vi "Fetch Multiple Record Multiple Channel (I16).vi"(5 "FIFO Type":enum16{"FPGA to Host FIFO (U64)", "Generic"}(ring), 7 "Timeout (s)":i32=5, 8 "error in":errorcluster, 10 "Records to Fetch":i32, 11 "FPGA VI Reference In":refnum<k20>) -> (0 "error out":errorcluster, 2 "Acquired Data":i16[][](array[numeric]), 3 "FPGA VI Reference Out":refnum<k20>, 4 "Elements Remaining":u32)   [LabVIEW 2011]
uses:
  <userlib>/FlexRIO Host Library/FlexRIO Host API/Acquire/Fetch/Fetch Acquired Data (U64).vi
  <vilib>/Utility/error.llb/Error Cluster From Error Code.vi
  <vilib>/rvi/errors/niLvFpgaAdjustHostInterfaceError.vi
  <vilib>/rvi/interface/nirviReadWriteControl/nirviReadWriteControl.xnode
  NiFpgaLv.dll
  <vilib>/rvi/interface/Simulation/niFpgaSimulationCallBeginRW.vi
  <userlib>/FlexRIO Host Library/FlexRIO Host Library (User).lvlib
  <userlib>/FlexRIO Host Library/FlexRIO Host API/Utility/memnoncopy.dll
panel:
  out "Data Acquired":i16[](array[numeric])
  out "Dummy Data":i16[](array[numeric])
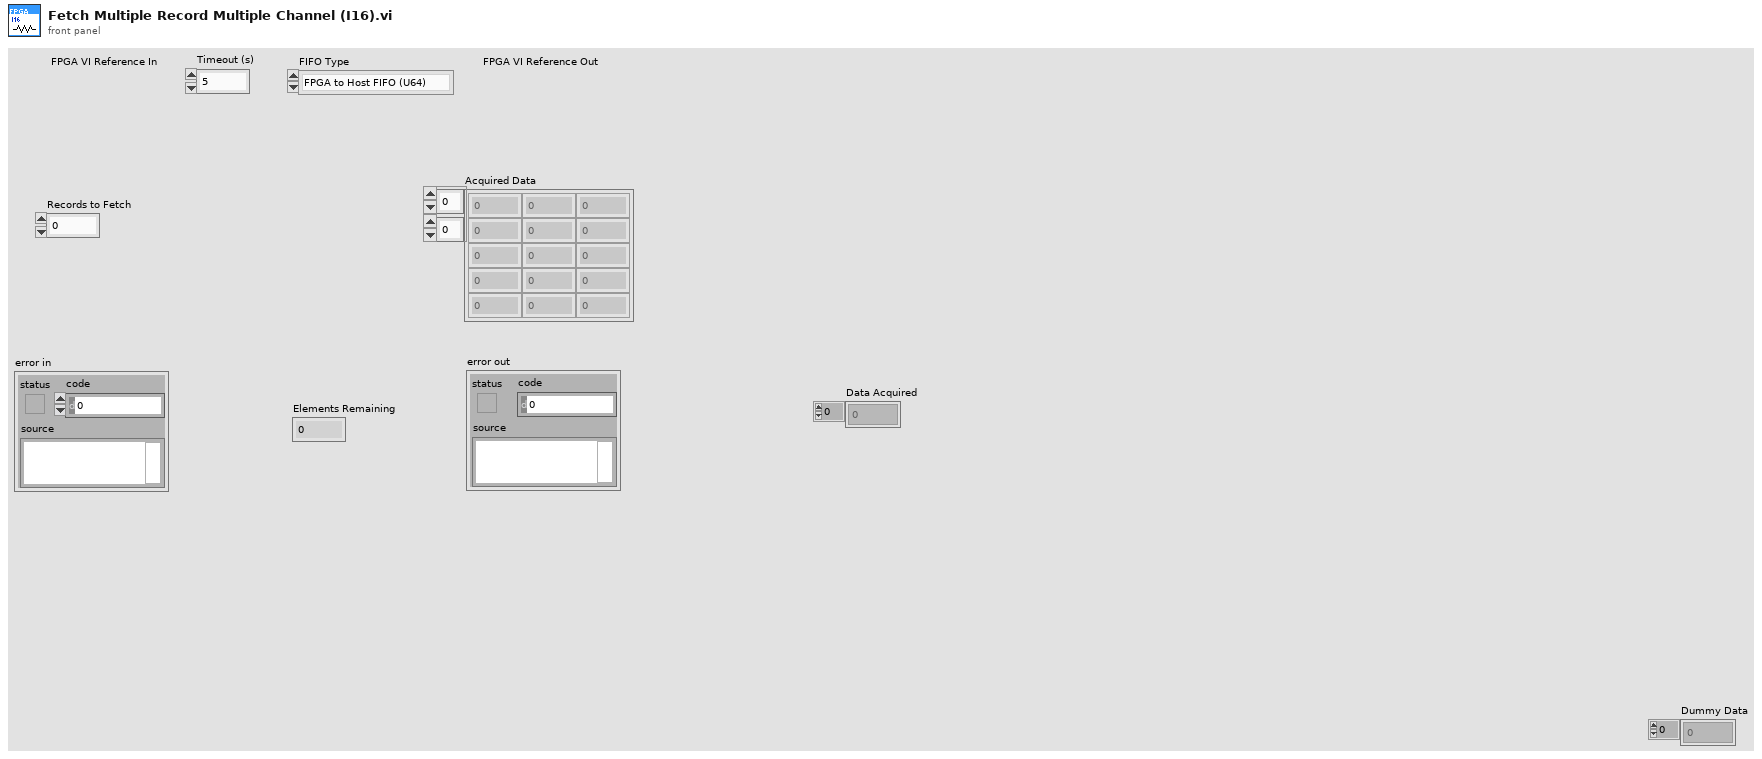
[diagram p1: front panel]
types:
  T1 = cluster{"Load Record Parameters?":bool, "Pre Trigger Samples":u16, "Samples per Record":u16, "Trigger Hold Off":u16, "Record Count":u16}
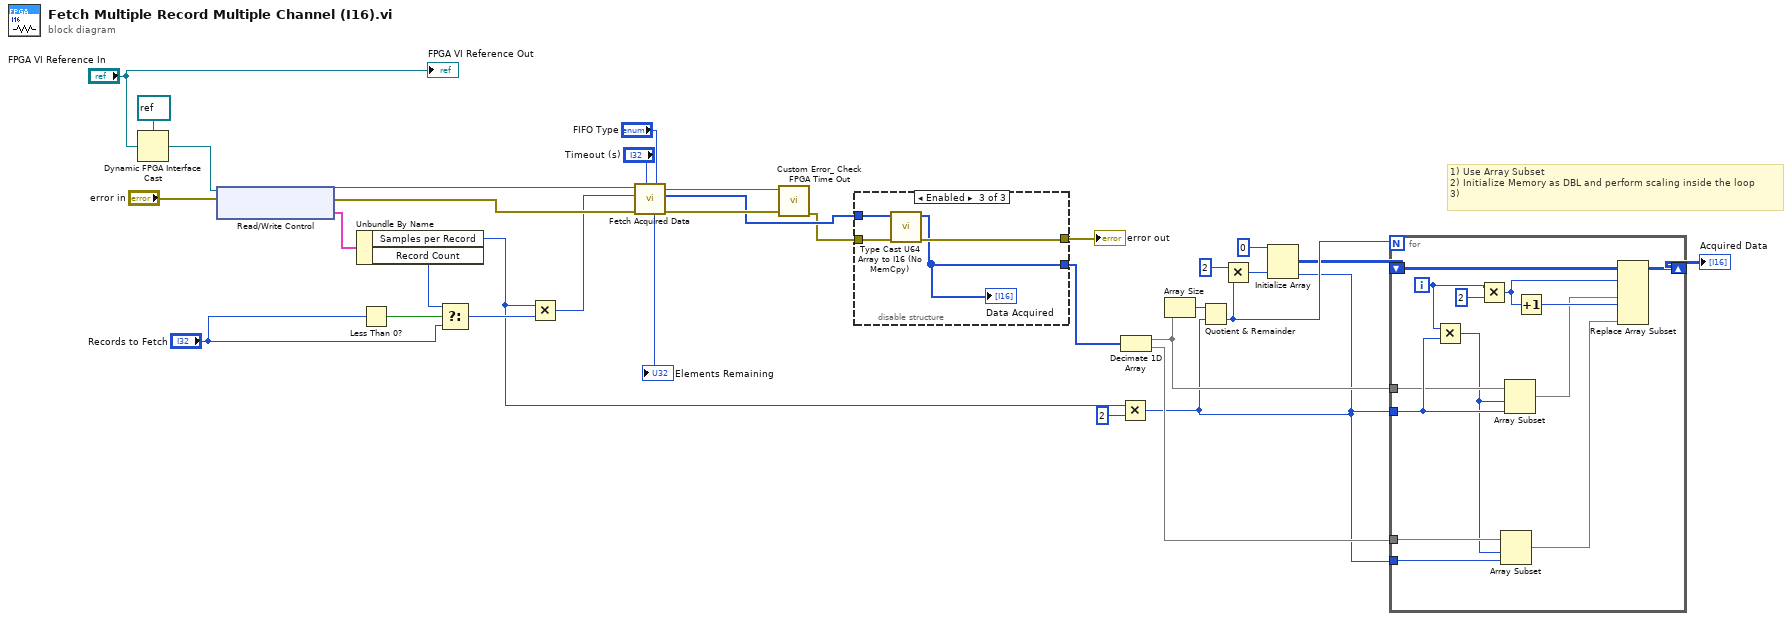
[diagram p0: block diagram]
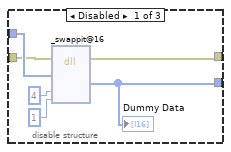
[diagram p2: hidden frame]
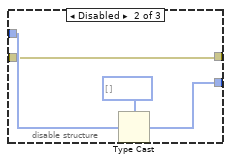
[diagram p3: hidden frame]
diagram:
  # "1) Use Array Subset\n2) Initialize Memory as DBL and perform scaling inside the loop\n3)"
  n1 = Dynamic FPGA Interface Cast(Session In=refnum<k20> refnum ("Type"), Type="FPGA VI Reference In") -> (Session Out=w30:refnum<k20>)
  n2 = xnode "Read/Write Control"("FPGA VI Reference In"=w30, "error in"="error in") -> ("FPGA VI Reference Out"=w25:refnum<k20>, "error out"=w24:errorcluster, "Record Parameters"=w29:T1)
  n3 = Unbundle By Name(w29) -> ("Samples per Record"=w18:u16, "Record Count"=w27:u16)
  n4 = Less Than 0?(x="Records to Fetch") -> (x < 0?=w28:bool)
  n5 = Select(t=w27, s=w28, f="Records to Fetch") -> (s? t:f=w19:i32)
  n6 = Multiply(x=w18, y=w19) -> (x*y=w23:i32)
  n7 = call-poly <userlib>:"Fetch Acquired Data.vi"("FIFO Type"="FIFO Type", "Timeout (s)"="Timeout (s)", "error out"=w24, "Samples"=w23, "FPGA Reference In"=w25) -> ("error out"=w13:errorcluster, "Data"=w4:u64[], "FPGA Reference Out"=w14:refnum<k20>, "Elements Remaining"=→"Elements Remaining":u32)  [unwired: 3 in]
  n8 = call <userlib>:"Custom Error_ Check FPGA Time Out.vi"("error in"=w13, "FPGA VI Reference In"=w14) -> ("error out"=w3:errorcluster)  [unwired: 8 in, 1 out]
  n9 = disable-structure shown="Enabled" {
    disable-tunnel: w4 -> [w37 w42 w47]
    disable-tunnel: w3 -> [w36 w40 w46]
    disable-tunnel: [w35 w40 w45] -> w2
    disable-tunnel: [w34 w41 w44] -> w1
    frame Disabled {
      n10 = dll-call lib="C:/Program Files (x86)/National Instruments/LabVIEW 2011/user.lib/FlexRIO Host Library/FlexRIO Host API/Utility/memnoncopy.dll" fn="_swappit@16"(error in=w36, "src"=w37, "upsize"=4, "downsize"=1) -> (error out=w35:errorcluster, "Dummy Data"=w34:i16[])  [unwired: 7 in, 1 out]
      "Dummy Data" <- w34
    }
    frame Disabled {
      n11 = Type Cast(type=i16[] [], x=w42) -> (*(type *) &x=w41:i16[])
    }
    frame Enabled {
      n12 = call <userlib>:"Type Cast U64 Array to I16 (No MemCpy).vi"("error in"=w46, "Input"=w47) -> ("error out"=w45:errorcluster, "Data Acquired"=w44:i16[])  [unwired: 8 in]
      "Data Acquired" <- w44
    }
  }
  "error out" <- w2
  n13 = Multiply(x=w18, y=u16 2) -> (x*y=w6:u16)
  n14 = Decimate 1D Array(w1) -> (w16:i16[], w7:i16[])
  n15 = Array Size(array=w16) -> (size(s)=w15:i32)
  n16 = Quotient & Remainder(x=w15, y=w6) -> (floor(x/y)=w10:i32)  [unwired: 1 out]
  n17 = Multiply(x=2, y=w10) -> (x*y=w11:i32)
  n18 = Initialize Array(i16 0 ("element"), w11, w6) -> (w8:i16[][])
  n19 = for {
    N: w10 -> [_]
    tunnel: w16 -> [w59]
    tunnel: w6 -> [w60]
    tunnel: w7 -> [w58]
    tunnel: w6 -> [w56]
    shift-right: [w54] -> w5
    shift-left: w8 -> [w55]
    i -> [w53]
    n20 = Multiply(x=w53, y=w60) -> (x*y=w57:i32)
    n21 = Multiply(x=w53, y=2) -> (x*y=w51:i32)
    n22 = Array Subset(array=w58, index=w57, length=w56) -> (w48:i16[])
    n23 = Array Subset(array=w59, index=w57, length=w60) -> (w49:i16[])
    n24 = Increment(x=w51) -> (x+1=w50:i32)
    n25 = Replace Array Subset(array=w55, new element #1=w49, index (row) #1=w51, new element #2=w48, index (row) #2=w50) -> (w54:i16[][])  [unwired: 2 in]
  }
  "Acquired Data" <- w5
  "FPGA VI Reference Out" <- "FPGA VI Reference In"
